vi "DataTypeColors.vi"() -> ()   [LabVIEW 2019]
panel:
  in  "BoolDataType":bool
  in  "StrDataType":string
  in  "IntDataType":u8
  in  "floatDataType":dbl
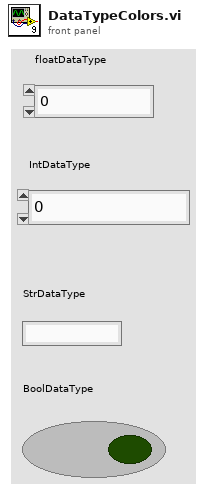
[diagram p1: front panel]
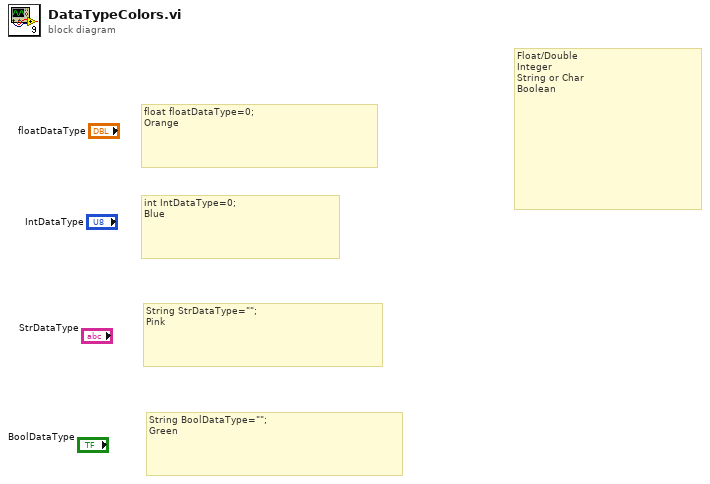
[diagram p0: block diagram]
diagram:
  # "String BoolDataType=\"\";\nGreen"
  # "String StrDataType=\"\";\nPink"
  # "int IntDataType=0;\nBlue"
  # "float floatDataType=0;\nOrange"
  # "Float/Double\nInteger\nString or Char\nBoolean"
